vi "ApplyLayoutToObject.vi"(5 "scaling settings":T1={"scaling factor"={"horizontal"=1.0, "vertical"=1.0}, "scale text"=FALSE} {"scaling factor"."vertical" min=0.0; "scaling factor"."horizontal" min=0.0}, 7 "properties to ignore":variant, 8 "error in (no error)":errorcluster, 10 "GObj Refnum":refnum<vi>, 11 "Path Control Layout in":refnum<class "Path Control Layout.lvclass">) -> (0 "error out":errorcluster, 3 "Path Control Layout out":refnum<class "Path Control Layout.lvclass">)   [LabVIEW 2012, in "NI_SE_Front Panel Layout.lvlib" / "Path Control Layout.lvclass"]
doc: "Apply layout information to the GObj Refnum."
uses:
  Path Control Layout.lvclass
  Scaling Factor_Options.ctl
  XY Scaling Factor.ctl
  Control Layout/Control Layout.lvclass
  Path Control Layout.lvclass/Path Control Layout.ctl
  Object Layout/Object Layout.lvclass/Object Layout.ctl
  Properties To Ignore.vi
  Set FP Object Size.vi
  NI_SE_Front Panel Layout.lvlib
  Object Layout/Object Layout.lvclass
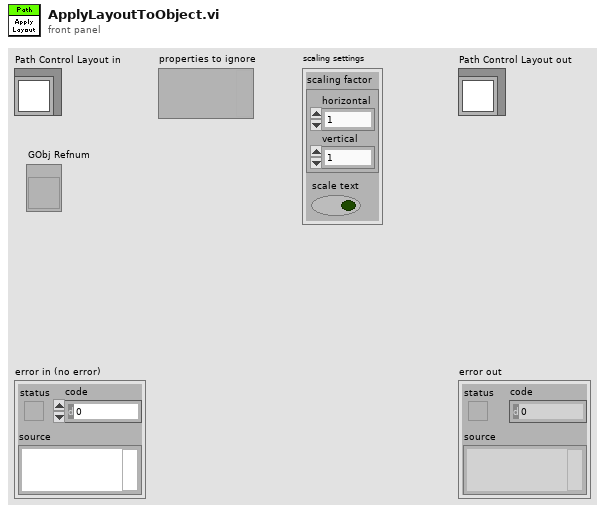
[diagram p1: front panel]
types:
  T1 = typedef "NI_SE_Front Panel Layout.lvlib/Scaling Factor_Options.ctl" = cluster{"scaling factor":T2, "scale text":bool}
  T2 = typedef "NI_SE_Front Panel Layout.lvlib/XY Scaling Factor.ctl" = cluster{"horizontal":dbl, "vertical":dbl}
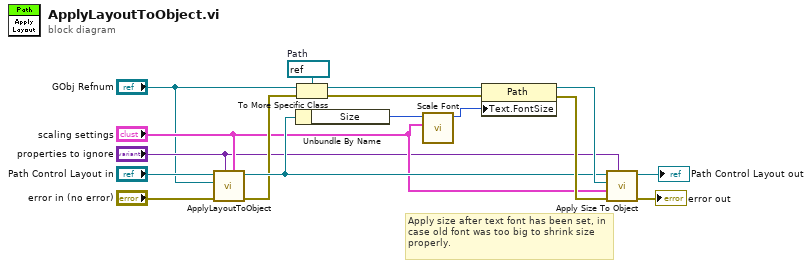
[diagram p0: block diagram]
diagram:
  w14 = refnum<vi> refnum  # Path
  # "Apply size after text font has been set, in case old font was too big to shrink size properly."
  n1 = call-parent "ApplyLayoutToObject.vi"("scaling settings"="scaling settings", "properties to ignore"="properties to ignore", "error in (no error)"="error in (no error)", "GObj Refnum"="GObj Refnum", "Control Layout in"="Path Control Layout in") -> ("error out"=w4:errorcluster, "Control Layout out"=w7:refnum<class "Path Control Layout.lvclass">)  [unwired: 5 in]
  n2 = Unbundle By Name(w7) -> ("Size"=w11:u16)
  n3 = To More Specific Class(target class=w14, reference="GObj Refnum", error in=w4) -> (specific class reference=w13:refnum<vi>, error out=w12:errorcluster)
  n4 = call "Scale Font.vi"("scaling settings"="scaling settings", "font size in"=w11) -> ("font size out"=w10:u16)  [unwired: 9 in]
  n5 = property class="Path"(reference=w13, error in=w12, "Text.FontSize"=w10) -> (reference out=w8:refnum<vi>, error out=w9:errorcluster)
  n6 = call "Apply Size To Object.vi"("properties to ignore"="properties to ignore", "error in (no error)"=w9, "scaling settings"="scaling settings", "GObj Refnum"=w8, "NI_SE_Object Layout in"=w7) -> ("error out"=→"error out":errorcluster, "NI_SE_Object Layout out"=→"Path Control Layout out":refnum<class "Path Control Layout.lvclass">)  [unwired: 5 in]
